vi "Z Stack Code.vi"() -> ()   [LabVIEW 2020]
uses:
  <vilib>/DAQmx/write.llb/DAQmx Write (Analog 1D Wfm NChan NSamp).vi
  <vilib>/DAQmx/create/channels.llb/DAQmx Create Channel (AO-Voltage-Basic).vi
  <vilib>/DAQmx/configure/timing.llb/DAQmx Timing (Use Waveform).vi
  <vilib>/DAQmx/miscellaneous.llb/DAQmx Fill In Error Info.vi
  <vilib>/Utility/file.llb/Read Delimited Spreadsheet (DBL).vi
  <vilib>/Analysis/polynomials.llb/Subtract Polynomials (DBL).vi
  <vilib>/measure/NI_MABase.lvlib
  <vilib>/Analysis/NI_AALPro.lvlib
panel:
  out "Waveform Graph":waveform(dbl)[](graph)=[{"t0"=timestamp(0 s since 1904-01-01), "dt"=0.0001, "Y"=array[10000 elements]}, {"t0"=timestamp(0 s since 1904-01-01), "dt"=0.0001, "Y"=array[10000 elements]}]
  out "dt":dbl=0.0001
  in  "file path (dialog if empty) 2":path=path "C:/Users/htm22/Downloads/Subtractfitvaluefromoutput.txt"
  out "x-y":dbl[](array[numeric])=[0.0, 0.0, 0.0, 0.0, 0.0, 0.0, 0.0, 0.0, 0.0, 0.0, 0.0, 0.0, 0.0, 0.0, 0.0, 0.0, 0.0, 0.0, 0.0, 0.0, 0.0, 0.0, 0.0, 0.0, 0.0, 0.0, 0.0, 0.0, 0.0, 0.0, 0.0, 0.0, 0.0, 0.0, 0.0, 0.0, 0.0, 0.0, 0.0, 0.0, 0.0, 0.0, 0.0, 0.0, 0.0, 0.0, 0.0, 0.0, 0.0, 0.0, 0.0, 0.0, 0.0, 0.0, 0.0, 0.0, 0.00936, -0.01208, 0.00648, -0.01496, 0.0036, 0.00216, -0.01928, -0.00072, -0.00216, -0.0036, -0.02504, 0.01352, 0.01208, -0.00936, 0.0092, 0.00776, -0.01368, -0.03512, -0.01656, -0.018, 0.00056, -0.00088, -0.02232, -0.00376, -0.0052, -0.02664, -0.02808, -0.00952, -0.01096, 0.0076, -0.01384, 0.00472, 0.00328, -0.01816, -0.0196, -0.02104, -0.02248, -0.00392, -0.00536, -0.0268, -0.00824, -0.00968, -0.01112, -0.01256, -0.014, 0.00456, 0.00312, 0.00168, 0.00024, -0.0212, -0.00264, -0.02408, -0.00552, -0.02696, -0.0084, -0.02984, 0.00872, 0.00728, -0.01416, -0.0356, -0.01704, 0.00152, 8e-05, -0.00136, -0.0028, -0.00424, -0.02568, -0.00712, -0.00856, -0.01, -0.01144, -0.03288, -0.03432, -0.01576, 0.0028, -0.01864, 0.01992, -0.02152, -0.02296, -0.0244, 0.01416, -0.00728, -0.00872, -0.01016, -0.0116, -0.01304, -0.01448, -0.01592, 0.00264, -0.0188, -0.02024, -0.00168, -0.00312, -0.04456, 0.014, -0.00744, -0.00888, 0.00968, -0.01176, 0.0068, -0.01464, -0.01608, -0.01752, 0.00104, -0.0004, -0.00184, -0.00328, -0.02472, -0.00616, -0.0076, -0.00904, -0.01048, -0.01192, -0.01336, -0.0148, -0.01624, -0.01768, -0.01912, -0.02056, -0.002, -0.00344, -0.02488, -0.00632, -0.02776, -0.0292, -0.03064, -0.01208, 0.00648, -0.01496, 0.0036, 0.00216, 0.00072, -0.00072, -0.02216, -0.0236, -0.00504, -0.00648, -0.00792, -0.00936, -0.0108, -0.01224, -0.01368, -0.01512, 0.00344, -0.018, 0.00056, -0.00088, -0.00232, -0.00376, -0.0052, -0.00664, -0.02808, -0.00952, 0.00904, -0.0124, -0.01384, -0.01528, -0.01672, -0.01816, -0.0196, -0.00104, -0.02248, -0.00392, 0.01464, -0.0068, -0.02824, 0.01032, -0.01112, 0.00744, -0.014, 0.00456, 0.00312, -0.01832, 0.00024, -0.0212, -0.02264, -0.00408, -0.00552, -0.02696, -0.0284, -0.00984, 0.00872, 0.00728, 0.00584, 0.0044, 0.00296, 0.00152, 8e-05, -0.02136, -0.0028, -0.02424, -0.00568, -0.00712, 0.01144, -0.01, -0.01144, -0.01288, 0.00568, -0.01576, -0.0172, 0.00136, -8e-05, -0.00152, -0.00296, 0.0156, -0.02584, -0.00728, -0.02872, -0.01016, -0.0116, -0.01304, 0.00552, -0.03592, -0.01736, -0.0188, -0.02024, -0.02168, -0.02312, -0.00456, -0.006, -0.00744, -0.00888, 0.00968, -0.01176, 0.0068, -0.01464, -0.01608, -0.01752, -0.01896, -0.0004, -0.00184, 0.01672, 0.01528, -0.00616, -0.0276, 0.01096, -0.01048, -0.01192, -0.01336, -0.0148, -0.01624, -0.01768, 0.00088, -0.02056, -0.022, -0.02344, -0.02488, 0.01368, -0.00776, -0.0092, -0.01064, -0.01208, 0.00648, -0.01496, -0.0364, -0.01784, 0.00072, -0.00072, -0.02216, -0.0036, -0.00504, -0.00648, -0.02792, -0.02936, 0.0092, 0.00776, 0.00632, -0.03512, 0.00344, -0.018, -0.01944, -0.00088, -0.00232, -0.00376, -0.0052, -0.02664, -0.00808, -0.00952, -0.01096, -0.0124, -0.01384, 0.00472, 0.00328, -0.01816, 0.0204, -0.00104, -0.00248, -0.00392, -0.00536, -0.0068, -0.02824, -0.02968, -0.01112, -0.01256, -0.014, -0.03544, 0.00312, 0.00168, 0.00024, -0.0012, -0.00264, -0.00408, -0.00552, -0.00696, -0.0084, 0.01016, -0.01128, -0.01272, 0.00584, -0.0156, -0.01704, 0.02152, 8e-05, -0.02136, -0.0028, -0.00424, -0.02568, -0.02712, 0.01144, 0.01, -0.01144, -0.01288, -0.01432, -0.01576, -0.0172, 0.00136, -0.02008, -0.00152, -0.02296, -0.0044, -0.02584, -0.00728, -0.02872, -0.01016, -0.0116, -0.01304, -0.01448, 0.00408, 0.00264, -0.0188, -0.02024, -0.00168, -0.02312, -0.02456, -0.006, -0.00744, -0.00888, -0.01032, -0.01176, -0.0132, -0.01464, -0.03608, 0.00248, 0.00104, -0.0204, 0.01816, -0.00328, -0.00472, -0.00616, -0.0076, -0.02904, -0.03048, -0.01192, -0.01336, -0.0148, 0.00376, -0.03768, -0.03912, -0.00056, -0.022, 0.01656, -0.00488, -0.00632, -0.00776, -0.0292, -0.01064, -0.01208, -0.01352, -0.01496, -0.0364, -0.01784, -0.01928, -0.02072, 0.01784, -0.0036, -0.02504, -0.00648, -0.00792, -0.02936, -0.0108, -0.01224, 0.00632, 0.00488, -0.01656, -0.038, 0.00056, -0.00088, -0.00232, -0.02376, -0.0052, -0.00664, -0.00808, -0.00952, -0.01096, -0.0324, -0.03384, -0.01528, -0.01672, -0.01816, -0.0196, -0.00104, -0.02248, -0.00392, -0.00536, -0.0068, -0.00824, -0.00968, 0.00888, -0.01256, -0.014, -0.01544, -0.01688, 0.00168, -0.01976, -0.0012, -0.00264, -0.00408, -0.02552, -0.00696, -0.0084, -0.00984, -0.01128, -0.01272, -0.01416, 0.0044, 0.00296, -0.01848, 8e-05, -0.00136, -0.0028, -0.02424, -0.00568, -0.00712, -0.00856, -0.01, -0.01144, -0.01288, -0.01432, -0.01576, 0.0028, -0.01864, -8e-05, -0.02152, -0.02296, -0.0044, -0.00584, -0.02728, -0.00872, -0.01016, -0.0116, -0.03304, -0.03448, -0.01592, -0.01736, -0.0188, -0.02024, -0.02168, -0.02312, -0.02456, -0.006, -0.02744, -0.00888, -0.03032, -0.01176, -0.0132, -0.01464, -0.01608, 0.00248, -0.01896, -0.0204, -0.02184, -0.02328, -0.00472, -0.00616, -0.0076, -0.00904, -0.01048, -0.01192, -0.01336, 0.0052, -0.01624, -0.01768, -0.01912, -0.02056, -0.022, -0.02344, -0.00488, -0.00632, -0.02776, -0.0292, 0.00936, -0.01208, -0.03352, 0.00504, 0.0036, -0.01784, -0.01928, -0.00072, -0.02216, -0.0236, -0.02504, -0.00648, -0.00792, -0.00936, -0.0308, -0.01224, 0.00632, -0.01512, -0.01656, -0.018, -0.01944, -0.02088, -0.00232, -0.00376, -0.0252, -0.00664, -0.00808, -0.00952, -0.01096, 0.0076, -0.01384, -0.01528, -0.01672, 0.00184, 0.0004, -0.00104, -0.02248, -0.02392, -0.02536, -0.0068, 0.01176, -0.00968, -0.01112, -0.01256, -0.014, -0.01544, 0.00312, -0.01832, -0.01976, -0.0212, -0.00264, -0.00408, -0.00552, -0.02696, -0.0084, -0.00984, 0.00872, -0.03272, 0.00584, -0.0156, -0.01704, -0.01848, -0.01992, -0.00136, -0.0028, -0.00424, -0.02568, -0.00712, -0.00856, -0.01, -0.01144, -0.01288, -0.01432, -0.01576, -0.0372, 0.00136, -0.02008, -0.02152, -0.02296, -0.0044, -0.02584, -0.00728, -0.00872, -0.03016, -0.0116, -0.03304, 0.00552, -0.03592, -0.01736, 0.0012, -0.00024, -0.02168, -0.02312, -0.02456, -0.006, -0.02744, -0.00888, -0.03032, -0.03176, -0.0332, -0.01464, -0.01608, -0.01752, 0.00104, -0.0004, -0.02184, -0.00328, -0.00472, -0.00616, -0.0076, -0.00904, -0.03048, -0.01192, -0.01336, -0.0148, -0.01624, -0.01768, -0.01912, -0.02056, -0.002, -0.02344, -0.00488, -0.00632, -0.02776, 0.0108, -0.01064, -0.01208, -0.01352, 0.00504, 0.0036, 0.00216, 0.00072, -0.02072, -0.02216, -0.0236, -0.02504, -0.00648, -0.00792, 0.01064, 0.0092, -0.01224, -0.01368, 0.00488, -0.01656, 0.002, 0.00056, -0.00088, -0.00232, -0.00376, -0.0252, -0.02664, -0.00808, -0.00952, -0.01096, -0.0124, -0.03384, 0.00472, -0.01672, -0.01816, -0.0196, -0.00104, -0.00248, 0.01608, -0.00536, -0.0068, -0.00824, -0.02968, 0.00888, 0.00744, -0.014, 0.00456, -0.01688, 0.00168, -0.01976, -0.0012, -0.00264, -0.00408, -0.00552, -0.00696, -0.0284, -0.00984, 0.00872, -0.01272, -0.01416, -0.0156, -0.01704, -0.01848, -0.01992, -0.00136, -0.0228, -0.00424, -0.00568, -0.00712, -0.00856, -0.01, -0.01144, -0.01288, -0.01432, 0.00424, 0.0028, 0.00136, -0.02008, -0.00152, -0.02296, -0.0044, -0.00584, -0.02728, -0.00872, -0.03016, -0.0316, -0.01304, 0.00552, -0.03592, -0.01736, -0.0188, -0.00024, -0.02168, -0.02312, 0.01544, -0.006, -0.00744, -0.02888, -0.01032, -0.01176, 0.0068, -0.01464, -0.01608, -0.01752, 0.00104, -0.0204, -0.00184, -0.00328, -0.00472, -0.02616, -0.0076, -0.02904, -0.01048, -0.01192, -0.01336, 0.0052, -0.01624, -0.01768, 0.00088, -0.02056, -0.022, -0.00344, -0.02488, -0.00632, -0.00776, -0.0092, 0.00936, -0.03208, 0.02648, -0.01496, 0.0036, -0.01784, -0.01928, -0.00072, -0.00216, -0.0036, -0.00504, -0.00648, -0.00792, -0.00936, 0.0092, -0.03224, -0.01368, -0.01512, -0.01656, 0.002, -0.01944, -0.02088, -0.00232, -0.00376, -0.0052, -0.00664, -0.00808, -0.00952, -0.01096, -0.0124, -0.01384, -0.01528, -0.01672, 0.00184, -0.0196, -0.04104, -0.02248, -0.00392, -0.00536, -0.0268, -0.00824, -0.00968, -0.01112, -0.01256, -0.014, 0.00456, -0.01688, -0.01832, -0.01976, -0.0012, -0.02264, -0.00408, -0.00552, 0.01304, 0.0116, -0.00984, -0.01128, -0.03272, -0.01416, -0.0156, 0.00296, 0.00152, 8e-05, -0.00136, -0.0228, -0.02424, -0.00568, -0.00712, -0.00856, -0.01, -0.01144, 0.00712, 0.00568, 0.00424, -0.0172, 0.00136, -0.02008, -0.02152, -0.02296, -0.0044, 0.01416, -0.00728, -0.02872, -0.01016, -0.0316, -0.01304, -0.01448, -0.01592, -0.01736, 0.0012, -0.02024, -0.02168, -0.00312, -0.00456, -0.006, -0.00744, 0.01112, -0.03032, -0.03176, -0.0332, -0.01464, -0.01608, -0.01752, 0.00104, -0.0004, -0.02184, -0.00328, 0.01528, -0.02616, -0.0076, -0.00904, -0.01048, -0.01192, -0.03336, -0.0148, -0.01624, -0.01768, 0.00088, -0.02056, -0.002, -0.00344, -0.02488, -0.02632, -0.02776, -0.0092, -0.01064, -0.01208, -0.01352, -0.01496, -0.0164, -0.01784, 0.00072, -0.00072, -0.04216, -0.0236, -0.00504, -0.00648, 0.01208, -0.00936, -0.0308, -0.03224, 0.00632, 0.00488, -0.01656, 0.002, 0.00056, -0.00088, -0.02232, -0.00376, -0.0052, -0.00664, -0.02808, -0.00952, -0.01096, -0.0124, -0.01384, -0.01528, -0.01672, -0.01816, 0.0004, -0.02104, -0.02248, -0.02392, -0.02536, -0.0068, -0.00824, -0.00968, 0.00888, -0.01256, -0.014, -0.01544, 0.00312, -0.03832, 0.00024, -0.0012, -0.00264, -0.02408, -0.00552, -0.02696, -0.0284, -0.00984, 0.00872, -0.01272, -0.01416, -0.0356, 0.00296, -0.01848, 8e-05, -0.00136, -0.0028, -0.02424, -0.02568, -0.00712, -0.00856]
  out "Signal - Fit":dbl[](graph)=[0.0, 0.0, 0.0, 0.0, 0.0, 0.0, 0.0, 0.0, 0.0, 0.0, 0.0, 0.0, 0.0, 0.0, 0.0, 0.0, 0.0, 0.0, 0.0, 0.0, 0.0, 0.0, 0.0, 0.0, 0.0, 0.0, 0.0, 0.0, 0.0, 0.0, 0.0, 0.0, 0.0, 0.0, 0.0, 0.0, 0.0, 0.0, 0.0, 0.0, 0.0, 0.0, 0.0, 0.0, 0.0, 0.0, 0.0, 0.0, 0.0, 0.0, 0.0, 0.0, 0.0, 0.0, 0.0, 0.0, 0.00936, -0.01208, 0.00648, -0.01496, 0.0036, 0.00216, -0.01928, -0.00072, -0.00216, -0.0036, -0.02504, 0.01352, 0.01208, -0.00936, 0.0092, 0.00776, -0.01368, -0.03512, -0.01656, -0.018, 0.00056, -0.00088, -0.02232, -0.00376, -0.0052, -0.02664, -0.02808, -0.00952, -0.01096, 0.0076, -0.01384, 0.00472, 0.00328, -0.01816, -0.0196, -0.02104, -0.02248, -0.00392, -0.00536, -0.0268, -0.00824, -0.00968, -0.01112, -0.01256, -0.014, 0.00456, 0.00312, 0.00168, 0.00024, -0.0212, -0.00264, -0.02408, -0.00552, -0.02696, -0.0084, -0.02984, 0.00872, 0.00728, -0.01416, -0.0356, -0.01704, 0.00152, 8e-05, -0.00136, -0.0028, -0.00424, -0.02568, -0.00712, -0.00856, -0.01, -0.01144, -0.03288, -0.03432, -0.01576, 0.0028, -0.01864, 0.01992, -0.02152, -0.02296, -0.0244, 0.01416, -0.00728, -0.00872, -0.01016, -0.0116, -0.01304, -0.01448, -0.01592, 0.00264, -0.0188, -0.02024, -0.00168, -0.00312, -0.04456, 0.014, -0.00744, -0.00888, 0.00968, -0.01176, 0.0068, -0.01464, -0.01608, -0.01752, 0.00104, -0.0004, -0.00184, -0.00328, -0.02472, -0.00616, -0.0076, -0.00904, -0.01048, -0.01192, -0.01336, -0.0148, -0.01624, -0.01768, -0.01912, -0.02056, -0.002, -0.00344, -0.02488, -0.00632, -0.02776, -0.0292, -0.03064, -0.01208, 0.00648, -0.01496, 0.0036, 0.00216, 0.00072, -0.00072, -0.02216, -0.0236, -0.00504, -0.00648, -0.00792, -0.00936, -0.0108, -0.01224, -0.01368, -0.01512, 0.00344, -0.018, 0.00056, -0.00088, -0.00232, -0.00376, -0.0052, -0.00664, -0.02808, -0.00952, 0.00904, -0.0124, -0.01384, -0.01528, -0.01672, -0.01816, -0.0196, -0.00104, -0.02248, -0.00392, 0.01464, -0.0068, -0.02824, 0.01032, -0.01112, 0.00744, -0.014, 0.00456, 0.00312, -0.01832, 0.00024, -0.0212, -0.02264, -0.00408, -0.00552, -0.02696, -0.0284, -0.00984, 0.00872, 0.00728, 0.00584, 0.0044, 0.00296, 0.00152, 8e-05, -0.02136, -0.0028, -0.02424, -0.00568, -0.00712, 0.01144, -0.01, -0.01144, -0.01288, 0.00568, -0.01576, -0.0172, 0.00136, -8e-05, -0.00152, -0.00296, 0.0156, -0.02584, -0.00728, -0.02872, -0.01016, -0.0116, -0.01304, 0.00552, -0.03592, -0.01736, -0.0188, -0.02024, -0.02168, -0.02312, -0.00456, -0.006, -0.00744, -0.00888, 0.00968, -0.01176, 0.0068, -0.01464, -0.01608, -0.01752, -0.01896, -0.0004, -0.00184, 0.01672, 0.01528, -0.00616, -0.0276, 0.01096, -0.01048, -0.01192, -0.01336, -0.0148, -0.01624, -0.01768, 0.00088, -0.02056, -0.022, -0.02344, -0.02488, 0.01368, -0.00776, -0.0092, -0.01064, -0.01208, 0.00648, -0.01496, -0.0364, -0.01784, 0.00072, -0.00072, -0.02216, -0.0036, -0.00504, -0.00648, -0.02792, -0.02936, 0.0092, 0.00776, 0.00632, -0.03512, 0.00344, -0.018, -0.01944, -0.00088, -0.00232, -0.00376, -0.0052, -0.02664, -0.00808, -0.00952, -0.01096, -0.0124, -0.01384, 0.00472, 0.00328, -0.01816, 0.0204, -0.00104, -0.00248, -0.00392, -0.00536, -0.0068, -0.02824, -0.02968, -0.01112, -0.01256, -0.014, -0.03544, 0.00312, 0.00168, 0.00024, -0.0012, -0.00264, -0.00408, -0.00552, -0.00696, -0.0084, 0.01016, -0.01128, -0.01272, 0.00584, -0.0156, -0.01704, 0.02152, 8e-05, -0.02136, -0.0028, -0.00424, -0.02568, -0.02712, 0.01144, 0.01, -0.01144, -0.01288, -0.01432, -0.01576, -0.0172, 0.00136, -0.02008, -0.00152, -0.02296, -0.0044, -0.02584, -0.00728, -0.02872, -0.01016, -0.0116, -0.01304, -0.01448, 0.00408, 0.00264, -0.0188, -0.02024, -0.00168, -0.02312, -0.02456, -0.006, -0.00744, -0.00888, -0.01032, -0.01176, -0.0132, -0.01464, -0.03608, 0.00248, 0.00104, -0.0204, 0.01816, -0.00328, -0.00472, -0.00616, -0.0076, -0.02904, -0.03048, -0.01192, -0.01336, -0.0148, 0.00376, -0.03768, -0.03912, -0.00056, -0.022, 0.01656, -0.00488, -0.00632, -0.00776, -0.0292, -0.01064, -0.01208, -0.01352, -0.01496, -0.0364, -0.01784, -0.01928, -0.02072, 0.01784, -0.0036, -0.02504, -0.00648, -0.00792, -0.02936, -0.0108, -0.01224, 0.00632, 0.00488, -0.01656, -0.038, 0.00056, -0.00088, -0.00232, -0.02376, -0.0052, -0.00664, -0.00808, -0.00952, -0.01096, -0.0324, -0.03384, -0.01528, -0.01672, -0.01816, -0.0196, -0.00104, -0.02248, -0.00392, -0.00536, -0.0068, -0.00824, -0.00968, 0.00888, -0.01256, -0.014, -0.01544, -0.01688, 0.00168, -0.01976, -0.0012, -0.00264, -0.00408, -0.02552, -0.00696, -0.0084, -0.00984, -0.01128, -0.01272, -0.01416, 0.0044, 0.00296, -0.01848, 8e-05, -0.00136, -0.0028, -0.02424, -0.00568, -0.00712, -0.00856, -0.01, -0.01144, -0.01288, -0.01432, -0.01576, 0.0028, -0.01864, -8e-05, -0.02152, -0.02296, -0.0044, -0.00584, -0.02728, -0.00872, -0.01016, -0.0116, -0.03304, -0.03448, -0.01592, -0.01736, -0.0188, -0.02024, -0.02168, -0.02312, -0.02456, -0.006, -0.02744, -0.00888, -0.03032, -0.01176, -0.0132, -0.01464, -0.01608, 0.00248, -0.01896, -0.0204, -0.02184, -0.02328, -0.00472, -0.00616, -0.0076, -0.00904, -0.01048, -0.01192, -0.01336, 0.0052, -0.01624, -0.01768, -0.01912, -0.02056, -0.022, -0.02344, -0.00488, -0.00632, -0.02776, -0.0292, 0.00936, -0.01208, -0.03352, 0.00504, 0.0036, -0.01784, -0.01928, -0.00072, -0.02216, -0.0236, -0.02504, -0.00648, -0.00792, -0.00936, -0.0308, -0.01224, 0.00632, -0.01512, -0.01656, -0.018, -0.01944, -0.02088, -0.00232, -0.00376, -0.0252, -0.00664, -0.00808, -0.00952, -0.01096, 0.0076, -0.01384, -0.01528, -0.01672, 0.00184, 0.0004, -0.00104, -0.02248, -0.02392, -0.02536, -0.0068, 0.01176, -0.00968, -0.01112, -0.01256, -0.014, -0.01544, 0.00312, -0.01832, -0.01976, -0.0212, -0.00264, -0.00408, -0.00552, -0.02696, -0.0084, -0.00984, 0.00872, -0.03272, 0.00584, -0.0156, -0.01704, -0.01848, -0.01992, -0.00136, -0.0028, -0.00424, -0.02568, -0.00712, -0.00856, -0.01, -0.01144, -0.01288, -0.01432, -0.01576, -0.0372, 0.00136, -0.02008, -0.02152, -0.02296, -0.0044, -0.02584, -0.00728, -0.00872, -0.03016, -0.0116, -0.03304, 0.00552, -0.03592, -0.01736, 0.0012, -0.00024, -0.02168, -0.02312, -0.02456, -0.006, -0.02744, -0.00888, -0.03032, -0.03176, -0.0332, -0.01464, -0.01608, -0.01752, 0.00104, -0.0004, -0.02184, -0.00328, -0.00472, -0.00616, -0.0076, -0.00904, -0.03048, -0.01192, -0.01336, -0.0148, -0.01624, -0.01768, -0.01912, -0.02056, -0.002, -0.02344, -0.00488, -0.00632, -0.02776, 0.0108, -0.01064, -0.01208, -0.01352, 0.00504, 0.0036, 0.00216, 0.00072, -0.02072, -0.02216, -0.0236, -0.02504, -0.00648, -0.00792, 0.01064, 0.0092, -0.01224, -0.01368, 0.00488, -0.01656, 0.002, 0.00056, -0.00088, -0.00232, -0.00376, -0.0252, -0.02664, -0.00808, -0.00952, -0.01096, -0.0124, -0.03384, 0.00472, -0.01672, -0.01816, -0.0196, -0.00104, -0.00248, 0.01608, -0.00536, -0.0068, -0.00824, -0.02968, 0.00888, 0.00744, -0.014, 0.00456, -0.01688, 0.00168, -0.01976, -0.0012, -0.00264, -0.00408, -0.00552, -0.00696, -0.0284, -0.00984, 0.00872, -0.01272, -0.01416, -0.0156, -0.01704, -0.01848, -0.01992, -0.00136, -0.0228, -0.00424, -0.00568, -0.00712, -0.00856, -0.01, -0.01144, -0.01288, -0.01432, 0.00424, 0.0028, 0.00136, -0.02008, -0.00152, -0.02296, -0.0044, -0.00584, -0.02728, -0.00872, -0.03016, -0.0316, -0.01304, 0.00552, -0.03592, -0.01736, -0.0188, -0.00024, -0.02168, -0.02312, 0.01544, -0.006, -0.00744, -0.02888, -0.01032, -0.01176, 0.0068, -0.01464, -0.01608, -0.01752, 0.00104, -0.0204, -0.00184, -0.00328, -0.00472, -0.02616, -0.0076, -0.02904, -0.01048, -0.01192, -0.01336, 0.0052, -0.01624, -0.01768, 0.00088, -0.02056, -0.022, -0.00344, -0.02488, -0.00632, -0.00776, -0.0092, 0.00936, -0.03208, 0.02648, -0.01496, 0.0036, -0.01784, -0.01928, -0.00072, -0.00216, -0.0036, -0.00504, -0.00648, -0.00792, -0.00936, 0.0092, -0.03224, -0.01368, -0.01512, -0.01656, 0.002, -0.01944, -0.02088, -0.00232, -0.00376, -0.0052, -0.00664, -0.00808, -0.00952, -0.01096, -0.0124, -0.01384, -0.01528, -0.01672, 0.00184, -0.0196, -0.04104, -0.02248, -0.00392, -0.00536, -0.0268, -0.00824, -0.00968, -0.01112, -0.01256, -0.014, 0.00456, -0.01688, -0.01832, -0.01976, -0.0012, -0.02264, -0.00408, -0.00552, 0.01304, 0.0116, -0.00984, -0.01128, -0.03272, -0.01416, -0.0156, 0.00296, 0.00152, 8e-05, -0.00136, -0.0228, -0.02424, -0.00568, -0.00712, -0.00856, -0.01, -0.01144, 0.00712, 0.00568, 0.00424, -0.0172, 0.00136, -0.02008, -0.02152, -0.02296, -0.0044, 0.01416, -0.00728, -0.02872, -0.01016, -0.0316, -0.01304, -0.01448, -0.01592, -0.01736, 0.0012, -0.02024, -0.02168, -0.00312, -0.00456, -0.006, -0.00744, 0.01112, -0.03032, -0.03176, -0.0332, -0.01464, -0.01608, -0.01752, 0.00104, -0.0004, -0.02184, -0.00328, 0.01528, -0.02616, -0.0076, -0.00904, -0.01048, -0.01192, -0.03336, -0.0148, -0.01624, -0.01768, 0.00088, -0.02056, -0.002, -0.00344, -0.02488, -0.02632, -0.02776, -0.0092, -0.01064, -0.01208, -0.01352, -0.01496, -0.0164, -0.01784, 0.00072, -0.00072, -0.04216, -0.0236, -0.00504, -0.00648, 0.01208, -0.00936, -0.0308, -0.03224, 0.00632, 0.00488, -0.01656, 0.002, 0.00056, -0.00088, -0.02232, -0.00376, -0.0052, -0.00664, -0.02808, -0.00952, -0.01096, -0.0124, -0.01384, -0.01528, -0.01672, -0.01816, 0.0004, -0.02104, -0.02248, -0.02392, -0.02536, -0.0068, -0.00824, -0.00968, 0.00888, -0.01256, -0.014, -0.01544, 0.00312, -0.03832, 0.00024, -0.0012, -0.00264, -0.02408, -0.00552, -0.02696, -0.0284, -0.00984, 0.00872, -0.01272, -0.01416, -0.0356, 0.00296, -0.01848, 8e-05, -0.00136, -0.0028, -0.02424, -0.02568, -0.00712, -0.00856]
  out "Array":dbl[](array[numeric])=[0.0, 0.001, 0.002, 0.003, 0.004, 0.005, 0.006, 0.007, 0.008, 0.009, 0.01, 0.011, 0.012, 0.013, 0.014, 0.015, 0.016, 0.017, 0.018, 0.019, 0.02, 0.021, 0.022, 0.023, 0.024, 0.025, 0.026, 0.027, 0.028, 0.029, 0.03, 0.031, 0.032, 0.033, 0.034, 0.035, 0.036, 0.037, 0.038, 0.039, 0.04, 0.041, 0.042, 0.043, 0.044, 0.045, 0.046, 0.047, 0.048, 0.049, 0.05, 0.051, 0.052, 0.053, 0.054, 0.055, 0.056, 0.057, 0.058, 0.059, 0.06, 0.061, 0.062, 0.063, 0.064, 0.065, 0.066, 0.067, 0.068, 0.069, 0.07, 0.071, 0.072, 0.073, 0.074, 0.075, 0.076, 0.077, 0.078, 0.079, 0.08, 0.081, 0.082, 0.083, 0.084, 0.085, 0.086, 0.087, 0.088, 0.089, 0.09, 0.091, 0.092, 0.093, 0.094, 0.095, 0.096, 0.097, 0.098, 0.099, 0.1, 0.101, 0.102, 0.103, 0.104, 0.105, 0.106, 0.107, 0.108, 0.109, 0.11, 0.111, 0.112, 0.113, 0.114, 0.115, 0.116, 0.117, 0.118, 0.119, 0.12, 0.121, 0.122, 0.123, 0.124, 0.125, 0.126, 0.127, 0.128, 0.129, 0.13, 0.131, 0.132, 0.133, 0.134, 0.135, 0.136, 0.137, 0.138, 0.139, 0.14, 0.141, 0.142, 0.143, 0.144, 0.145, 0.146, 0.147, 0.148, 0.149, 0.15, 0.151, 0.152, 0.153, 0.154, 0.155, 0.156, 0.157, 0.158, 0.159, 0.16, 0.161, 0.162, 0.163, 0.164, 0.165, 0.166, 0.167, 0.168, 0.169, 0.17, 0.171, 0.172, 0.173, 0.174, 0.175, 0.176, 0.177, 0.178, 0.179, 0.18, 0.181, 0.182, 0.183, 0.184, 0.185, 0.186, 0.187, 0.188, 0.189, 0.19, 0.191, 0.192, 0.193, 0.194, 0.195, 0.196, 0.197, 0.198, 0.199, 0.2, 0.201, 0.202, 0.203, 0.204, 0.205, 0.206, 0.207, 0.208, 0.209, 0.21, 0.211, 0.212, 0.213, 0.214, 0.215, 0.216, 0.217, 0.218, 0.219, 0.22, 0.221, 0.222, 0.223, 0.224, 0.225, 0.226, 0.227, 0.228, 0.229, 0.23, 0.231, 0.232, 0.233, 0.234, 0.235, 0.236, 0.237, 0.238, 0.239, 0.24, 0.241, 0.242, 0.243, 0.244, 0.245, 0.246, 0.247, 0.248, 0.249, 0.25, 0.251, 0.252, 0.253, 0.254, 0.255, 0.256, 0.257, 0.258, 0.259, 0.26, 0.261, 0.262, 0.263, 0.264, 0.265, 0.266, 0.267, 0.268, 0.269, 0.27, 0.271, 0.272, 0.273, 0.274, 0.275, 0.276, 0.277, 0.278, 0.279, 0.28, 0.281, 0.282, 0.283, 0.284, 0.285, 0.286, 0.287, 0.288, 0.289, 0.29, 0.291, 0.292, 0.293, 0.294, 0.295, 0.296, 0.297, 0.298, 0.299, 0.3, 0.301, 0.302, 0.303, 0.304, 0.305, 0.306, 0.307, 0.308, 0.309, 0.31, 0.311, 0.312, 0.313, 0.314, 0.315, 0.316, 0.317, 0.318, 0.319, 0.32, 0.321, 0.322, 0.323, 0.324, 0.325, 0.326, 0.327, 0.328, 0.329, 0.33, 0.331, 0.332, 0.333, 0.334, 0.335, 0.336, 0.337, 0.338, 0.339, 0.34, 0.341, 0.342, 0.343, 0.344, 0.345, 0.346, 0.347, 0.348, 0.349, 0.35, 0.351, 0.352, 0.353, 0.354, 0.355, 0.356, 0.357, 0.358, 0.359, 0.36, 0.361, 0.362, 0.363, 0.364, 0.365, 0.366, 0.367, 0.368, 0.369, 0.37, 0.371, 0.372, 0.373, 0.374, 0.375, 0.376, 0.377, 0.378, 0.379, 0.38, 0.381, 0.382, 0.383, 0.384, 0.385, 0.386, 0.387, 0.388, 0.389, 0.39, 0.391, 0.392, 0.393, 0.394, 0.395, 0.396, 0.397, 0.398, 0.399, 0.4, 0.401, 0.402, 0.403, 0.404, 0.405, 0.406, 0.407, 0.408, 0.409, 0.41, 0.411, 0.412, 0.413, 0.414, 0.415, 0.416, 0.417, 0.418, 0.419, 0.42, 0.421, 0.422, 0.423, 0.424, 0.425, 0.426, 0.427, 0.428, 0.429, 0.43, 0.431, 0.432, 0.433, 0.434, 0.435, 0.436, 0.437, 0.438, 0.439, 0.44, 0.441, 0.442, 0.443, 0.444, 0.445, 0.446, 0.447, 0.448, 0.449, 0.45, 0.451, 0.452, 0.453, 0.454, 0.455, 0.456, 0.457, 0.458, 0.459, 0.46, 0.461, 0.462, 0.463, 0.464, 0.465, 0.466, 0.467, 0.468, 0.469, 0.47, 0.471, 0.472, 0.473, 0.474, 0.475, 0.476, 0.477, 0.478, 0.479, 0.48, 0.481, 0.482, 0.483, 0.484, 0.485, 0.486, 0.487, 0.488, 0.489, 0.49, 0.491, 0.492, 0.493, 0.494, 0.495, 0.496, 0.497, 0.498, 0.499, 0.5, 0.501, 0.502, 0.503, 0.504, 0.505, 0.506, 0.507, 0.508, 0.509, 0.51, 0.511, 0.512, 0.513, 0.514, 0.515, 0.516, 0.517, 0.518, 0.519, 0.52, 0.521, 0.522, 0.523, 0.524, 0.525, 0.526, 0.527, 0.528, 0.529, 0.53, 0.531, 0.532, 0.533, 0.534, 0.535, 0.536, 0.537, 0.538, 0.539, 0.54, 0.541, 0.542, 0.543, 0.544, 0.545, 0.546, 0.547, 0.548, 0.549, 0.55, 0.551, 0.552, 0.553, 0.554, 0.555, 0.556, 0.557, 0.558, 0.559, 0.56, 0.561, 0.562, 0.563, 0.564, 0.565, 0.566, 0.567, 0.568, 0.569, 0.57, 0.571, 0.572, 0.573, 0.574, 0.575, 0.576, 0.577, 0.578, 0.579, 0.58, 0.581, 0.582, 0.583, 0.584, 0.585, 0.586, 0.587, 0.588, 0.589, 0.59, 0.591, 0.592, 0.593, 0.594, 0.595, 0.596, 0.597, 0.598, 0.599, 0.6, 0.601, 0.602, 0.603, 0.604, 0.605, 0.606, 0.607, 0.608, 0.609, 0.61, 0.611, 0.612, 0.613, 0.614, 0.615, 0.616, 0.617, 0.618, 0.619, 0.62, 0.621, 0.622, 0.623, 0.624, 0.625, 0.626, 0.627, 0.628, 0.629, 0.63, 0.631, 0.632, 0.633, 0.634, 0.635, 0.636, 0.637, 0.638, 0.639, 0.64, 0.641, 0.642, 0.643, 0.644, 0.645, 0.646, 0.647, 0.648, 0.649, 0.65, 0.651, 0.652, 0.653, 0.654, 0.655, 0.656, 0.657, 0.658, 0.659, 0.66, 0.661, 0.662, 0.663, 0.664, 0.665, 0.666, 0.667, 0.668, 0.669, 0.67, 0.671, 0.672, 0.673, 0.674, 0.675, 0.676, 0.677, 0.678, 0.679, 0.68, 0.681, 0.682, 0.683, 0.684, 0.685, 0.686, 0.687, 0.688, 0.689, 0.69, 0.691, 0.692, 0.693, 0.694, 0.695, 0.696, 0.697, 0.698, 0.699, 0.7, 0.701, 0.702, 0.703, 0.704, 0.705, 0.706, 0.707, 0.708, 0.709, 0.71, 0.711, 0.712, 0.713, 0.714, 0.715, 0.716, 0.717, 0.718, 0.719, 0.72, 0.721, 0.722, 0.723, 0.724, 0.725, 0.726, 0.727, 0.728, 0.729, 0.73, 0.731, 0.732, 0.733, 0.734, 0.735, 0.736, 0.737, 0.738, 0.739, 0.74, 0.741, 0.742, 0.743, 0.744, 0.745, 0.746, 0.747, 0.748, 0.749, 0.75, 0.751, 0.752, 0.753, 0.754, 0.755, 0.756, 0.757, 0.758, 0.759, 0.76, 0.761, 0.762, 0.763, 0.764, 0.765, 0.766, 0.767, 0.768, 0.769, 0.77, 0.771, 0.772, 0.773, 0.774, 0.775, 0.776, 0.777, 0.778, 0.779, 0.78, 0.781, 0.782, 0.783, 0.784, 0.785, 0.786, 0.787, 0.788, 0.789, 0.79, 0.791, 0.792, 0.793, 0.794, 0.795, 0.796, 0.797, 0.798, 0.799, 0.8, 0.801, 0.802, 0.803, 0.804, 0.805, 0.806, 0.807, 0.808, 0.809, 0.81, 0.811, 0.812, 0.813, 0.814, 0.815, 0.816, 0.817, 0.818, 0.819, 0.82, 0.821, 0.822, 0.823, 0.824, 0.825, 0.826, 0.827, 0.828, 0.829, 0.83, 0.831, 0.832, 0.833, 0.834, 0.835, 0.836, 0.837, 0.838, 0.839, 0.84, 0.841, 0.842, 0.843, 0.844, 0.845, 0.846, 0.847, 0.848, 0.849, 0.85, 0.851, 0.852, 0.853, 0.854, 0.855, 0.856, 0.857, 0.858, 0.859, 0.86, 0.861, 0.862, 0.863, 0.864, 0.865, 0.866, 0.867, 0.868, 0.869, 0.87, 0.871, 0.872, 0.873, 0.874, 0.875, 0.876, 0.877, 0.878, 0.879, 0.88, 0.881, 0.882, 0.883, 0.884, 0.885, 0.886, 0.887, 0.888, 0.889, 0.89, 0.891, 0.892, 0.893, 0.894, 0.895, 0.896, 0.897, 0.898, 0.899, 0.9, 0.901, 0.902, 0.903, 0.904, 0.905, 0.906, 0.907, 0.908, 0.909, 0.91, 0.911, 0.912, 0.913, 0.914, 0.915, 0.916, 0.917, 0.918, 0.919, 0.92, 0.921, 0.922, 0.923, 0.924, 0.925, 0.926, 0.927, 0.928, 0.929, 0.93, 0.931, 0.932, 0.933, 0.934, 0.935, 0.936, 0.937, 0.938, 0.939, 0.94, 0.941, 0.942, 0.943, 0.944, 0.945, 0.946, 0.947, 0.948, 0.949, 0.95, 0.951, 0.952, 0.953, 0.954, 0.955, 0.956, 0.957, 0.958, 0.959, 0.96, 0.961, 0.962, 0.963, 0.964, 0.965, 0.966, 0.967, 0.968, 0.969, 0.97, 0.971, 0.972, 0.973, 0.974, 0.975, 0.976, 0.977, 0.978, 0.979, 0.98, 0.981, 0.982, 0.983, 0.984, 0.985, 0.986, 0.987, 0.988, 0.989, 0.99, 0.991, 0.992, 0.993, 0.994, 0.995, 0.996, 0.997, 0.998, 0.999]
  out "all rows 2":dbl[][](array[numeric])=[[0.0], [0.0], [0.0], [0.0], [0.0], [0.0], [0.0], [0.0], [0.0], [0.0], [0.0], [0.0], [0.0], [0.0], [0.0], [0.0], [0.0], [0.0], [0.0], [0.0], [0.0], [0.0], [0.0], [0.0], [0.0], [0.0], [0.0], [0.0], [0.0], [0.0], [0.0], [0.0], [0.0], [0.0], [0.0], [0.0], [0.0], [0.0], [0.0], [0.0], [0.0], [0.0], [0.0], [0.0], [0.0], [0.0], [0.0], [0.0], [0.0], [0.0], [0.0], [0.0], [0.0], [0.0], [0.0], [0.0], [0.00936], [-0.01208], [0.00648], [-0.01496], [0.0036], [0.00216], [-0.01928], [-0.00072], [-0.00216], [-0.0036], [-0.02504], [0.01352], [0.01208], [-0.00936], [0.0092], [0.00776], [-0.01368], [-0.03512], [-0.01656], [-0.018], [0.00056], [-0.00088], [-0.02232], [-0.00376], [-0.0052], [-0.02664], [-0.02808], [-0.00952], [-0.01096], [0.0076], [-0.01384], [0.00472], [0.00328], [-0.01816], [-0.0196], [-0.02104], [-0.02248], [-0.00392], [-0.00536], [-0.0268], [-0.00824], [-0.00968], [-0.01112], [-0.01256], [-0.014], [0.00456], [0.00312], [0.00168], [0.00024], [-0.0212], [-0.00264], [-0.02408], [-0.00552], [-0.02696], [-0.0084], [-0.02984], [0.00872], [0.00728], [-0.01416], [-0.0356], [-0.01704], [0.00152], [8e-05], [-0.00136], [-0.0028], [-0.00424], [-0.02568], [-0.00712], [-0.00856], [-0.01], [-0.01144], [-0.03288], [-0.03432], [-0.01576], [0.0028], [-0.01864], [0.01992], [-0.02152], [-0.02296], [-0.0244], [0.01416], [-0.00728], [-0.00872], [-0.01016], [-0.0116], [-0.01304], [-0.01448], [-0.01592], [0.00264], [-0.0188], [-0.02024], [-0.00168], [-0.00312], [-0.04456], [0.014], [-0.00744], [-0.00888], [0.00968], [-0.01176], [0.0068], [-0.01464], [-0.01608], [-0.01752], [0.00104], [-0.0004], [-0.00184], [-0.00328], [-0.02472], [-0.00616], [-0.0076], [-0.00904], [-0.01048], [-0.01192], [-0.01336], [-0.0148], [-0.01624], [-0.01768], [-0.01912], [-0.02056], [-0.002], [-0.00344], [-0.02488], [-0.00632], [-0.02776], [-0.0292], [-0.03064], [-0.01208], [0.00648], [-0.01496], [0.0036], [0.00216], [0.00072], [-0.00072], [-0.02216], [-0.0236], [-0.00504], [-0.00648], [-0.00792], [-0.00936], [-0.0108], [-0.01224], [-0.01368], [-0.01512], [0.00344], [-0.018], [0.00056], [-0.00088], [-0.00232], [-0.00376], [-0.0052], [-0.00664], [-0.02808], [-0.00952], [0.00904], [-0.0124], [-0.01384], [-0.01528], [-0.01672], [-0.01816], [-0.0196], [-0.00104], [-0.02248], [-0.00392], [0.01464], [-0.0068], [-0.02824], [0.01032], [-0.01112], [0.00744], [-0.014], [0.00456], [0.00312], [-0.01832], [0.00024], [-0.0212], [-0.02264], [-0.00408], [-0.00552], [-0.02696], [-0.0284], [-0.00984], [0.00872], [0.00728], [0.00584], [0.0044], [0.00296], [0.00152], [8e-05], [-0.02136], [-0.0028], [-0.02424], [-0.00568], [-0.00712], [0.01144], [-0.01], [-0.01144], [-0.01288], [0.00568], [-0.01576], [-0.0172], [0.00136], [-8e-05], [-0.00152], [-0.00296], [0.0156], [-0.02584], [-0.00728], [-0.02872], [-0.01016], [-0.0116], [-0.01304], [0.00552], [-0.03592], [-0.01736], [-0.0188], [-0.02024], [-0.02168], [-0.02312], [-0.00456], [-0.006], [-0.00744], [-0.00888], [0.00968], [-0.01176], [0.0068], [-0.01464], [-0.01608], [-0.01752], [-0.01896], [-0.0004], [-0.00184], [0.01672], [0.01528], [-0.00616], [-0.0276], [0.01096], [-0.01048], [-0.01192], [-0.01336], [-0.0148], [-0.01624], [-0.01768], [0.00088], [-0.02056], [-0.022], [-0.02344], [-0.02488], [0.01368], [-0.00776], [-0.0092], [-0.01064], [-0.01208], [0.00648], [-0.01496], [-0.0364], [-0.01784], [0.00072], [-0.00072], [-0.02216], [-0.0036], [-0.00504], [-0.00648], [-0.02792], [-0.02936], [0.0092], [0.00776], [0.00632], [-0.03512], [0.00344], [-0.018], [-0.01944], [-0.00088], [-0.00232], [-0.00376], [-0.0052], [-0.02664], [-0.00808], [-0.00952], [-0.01096], [-0.0124], [-0.01384], [0.00472], [0.00328], [-0.01816], [0.0204], [-0.00104], [-0.00248], [-0.00392], [-0.00536], [-0.0068], [-0.02824], [-0.02968], [-0.01112], [-0.01256], [-0.014], [-0.03544], [0.00312], [0.00168], [0.00024], [-0.0012], [-0.00264], [-0.00408], [-0.00552], [-0.00696], [-0.0084], [0.01016], [-0.01128], [-0.01272], [0.00584], [-0.0156], [-0.01704], [0.02152], [8e-05], [-0.02136], [-0.0028], [-0.00424], [-0.02568], [-0.02712], [0.01144], [0.01], [-0.01144], [-0.01288], [-0.01432], [-0.01576], [-0.0172], [0.00136], [-0.02008], [-0.00152], [-0.02296], [-0.0044], [-0.02584], [-0.00728], [-0.02872], [-0.01016], [-0.0116], [-0.01304], [-0.01448], [0.00408], [0.00264], [-0.0188], [-0.02024], [-0.00168], [-0.02312], [-0.02456], [-0.006], [-0.00744], [-0.00888], [-0.01032], [-0.01176], [-0.0132], [-0.01464], [-0.03608], [0.00248], [0.00104], [-0.0204], [0.01816], [-0.00328], [-0.00472], [-0.00616], [-0.0076], [-0.02904], [-0.03048], [-0.01192], [-0.01336], [-0.0148], [0.00376], [-0.03768], [-0.03912], [-0.00056], [-0.022], [0.01656], [-0.00488], [-0.00632], [-0.00776], [-0.0292], [-0.01064], [-0.01208], [-0.01352], [-0.01496], [-0.0364], [-0.01784], [-0.01928], [-0.02072], [0.01784], [-0.0036], [-0.02504], [-0.00648], [-0.00792], [-0.02936], [-0.0108], [-0.01224], [0.00632], [0.00488], [-0.01656], [-0.038], [0.00056], [-0.00088], [-0.00232], [-0.02376], [-0.0052], [-0.00664], [-0.00808], [-0.00952], [-0.01096], [-0.0324], [-0.03384], [-0.01528], [-0.01672], [-0.01816], [-0.0196], [-0.00104], [-0.02248], [-0.00392], [-0.00536], [-0.0068], [-0.00824], [-0.00968], [0.00888], [-0.01256], [-0.014], [-0.01544], [-0.01688], [0.00168], [-0.01976], [-0.0012], [-0.00264], [-0.00408], [-0.02552], [-0.00696], [-0.0084], [-0.00984], [-0.01128], [-0.01272], [-0.01416], [0.0044], [0.00296], [-0.01848], [8e-05], [-0.00136], [-0.0028], [-0.02424], [-0.00568], [-0.00712], [-0.00856], [-0.01], [-0.01144], [-0.01288], [-0.01432], [-0.01576], [0.0028], [-0.01864], [-8e-05], [-0.02152], [-0.02296], [-0.0044], [-0.00584], [-0.02728], [-0.00872], [-0.01016], [-0.0116], [-0.03304], [-0.03448], [-0.01592], [-0.01736], [-0.0188], [-0.02024], [-0.02168], [-0.02312], [-0.02456], [-0.006], [-0.02744], [-0.00888], [-0.03032], [-0.01176], [-0.0132], [-0.01464], [-0.01608], [0.00248], [-0.01896], [-0.0204], [-0.02184], [-0.02328], [-0.00472], [-0.00616], [-0.0076], [-0.00904], [-0.01048], [-0.01192], [-0.01336], [0.0052], [-0.01624], [-0.01768], [-0.01912], [-0.02056], [-0.022], [-0.02344], [-0.00488], [-0.00632], [-0.02776], [-0.0292], [0.00936], [-0.01208], [-0.03352], [0.00504], [0.0036], [-0.01784], [-0.01928], [-0.00072], [-0.02216], [-0.0236], [-0.02504], [-0.00648], [-0.00792], [-0.00936], [-0.0308], [-0.01224], [0.00632], [-0.01512], [-0.01656], [-0.018], [-0.01944], [-0.02088], [-0.00232], [-0.00376], [-0.0252], [-0.00664], [-0.00808], [-0.00952], [-0.01096], [0.0076], [-0.01384], [-0.01528], [-0.01672], [0.00184], [0.0004], [-0.00104], [-0.02248], [-0.02392], [-0.02536], [-0.0068], [0.01176], [-0.00968], [-0.01112], [-0.01256], [-0.014], [-0.01544], [0.00312], [-0.01832], [-0.01976], [-0.0212], [-0.00264], [-0.00408], [-0.00552], [-0.02696], [-0.0084], [-0.00984], [0.00872], [-0.03272], [0.00584], [-0.0156], [-0.01704], [-0.01848], [-0.01992], [-0.00136], [-0.0028], [-0.00424], [-0.02568], [-0.00712], [-0.00856], [-0.01], [-0.01144], [-0.01288], [-0.01432], [-0.01576], [-0.0372], [0.00136], [-0.02008], [-0.02152], [-0.02296], [-0.0044], [-0.02584], [-0.00728], [-0.00872], [-0.03016], [-0.0116], [-0.03304], [0.00552], [-0.03592], [-0.01736], [0.0012], [-0.00024], [-0.02168], [-0.02312], [-0.02456], [-0.006], [-0.02744], [-0.00888], [-0.03032], [-0.03176], [-0.0332], [-0.01464], [-0.01608], [-0.01752], [0.00104], [-0.0004], [-0.02184], [-0.00328], [-0.00472], [-0.00616], [-0.0076], [-0.00904], [-0.03048], [-0.01192], [-0.01336], [-0.0148], [-0.01624], [-0.01768], [-0.01912], [-0.02056], [-0.002], [-0.02344], [-0.00488], [-0.00632], [-0.02776], [0.0108], [-0.01064], [-0.01208], [-0.01352], [0.00504], [0.0036], [0.00216], [0.00072], [-0.02072], [-0.02216], [-0.0236], [-0.02504], [-0.00648], [-0.00792], [0.01064], [0.0092], [-0.01224], [-0.01368], [0.00488], [-0.01656], [0.002], [0.00056], [-0.00088], [-0.00232], [-0.00376], [-0.0252], [-0.02664], [-0.00808], [-0.00952], [-0.01096], [-0.0124], [-0.03384], [0.00472], [-0.01672], [-0.01816], [-0.0196], [-0.00104], [-0.00248], [0.01608], [-0.00536], [-0.0068], [-0.00824], [-0.02968], [0.00888], [0.00744], [-0.014], [0.00456], [-0.01688], [0.00168], [-0.01976], [-0.0012], [-0.00264], [-0.00408], [-0.00552], [-0.00696], [-0.0284], [-0.00984], [0.00872], [-0.01272], [-0.01416], [-0.0156], [-0.01704], [-0.01848], [-0.01992], [-0.00136], [-0.0228], [-0.00424], [-0.00568], [-0.00712], [-0.00856], [-0.01], [-0.01144], [-0.01288], [-0.01432], [0.00424], [0.0028], [0.00136], [-0.02008], [-0.00152], [-0.02296], [-0.0044], [-0.00584], [-0.02728], [-0.00872], [-0.03016], [-0.0316], [-0.01304], [0.00552], [-0.03592], [-0.01736], [-0.0188], [-0.00024], [-0.02168], [-0.02312], [0.01544], [-0.006], [-0.00744], [-0.02888], [-0.01032], [-0.01176], [0.0068], [-0.01464], [-0.01608], [-0.01752], [0.00104], [-0.0204], [-0.00184], [-0.00328], [-0.00472], [-0.02616], [-0.0076], [-0.02904], [-0.01048], [-0.01192], [-0.01336], [0.0052], [-0.01624], [-0.01768], [0.00088], [-0.02056], [-0.022], [-0.00344], [-0.02488], [-0.00632], [-0.00776], [-0.0092], [0.00936], [-0.03208], [0.02648], [-0.01496], [0.0036], [-0.01784], [-0.01928], [-0.00072], [-0.00216], [-0.0036], [-0.00504], [-0.00648], [-0.00792], [-0.00936], [0.0092], [-0.03224], [-0.01368], [-0.01512], [-0.01656], [0.002], [-0.01944], [-0.02088], [-0.00232], [-0.00376], [-0.0052], [-0.00664], [-0.00808], [-0.00952], [-0.01096], [-0.0124], [-0.01384], [-0.01528], [-0.01672], [0.00184], [-0.0196], [-0.04104], [-0.02248], [-0.00392], [-0.00536], [-0.0268], [-0.00824], [-0.00968], [-0.01112], [-0.01256], [-0.014], [0.00456], [-0.01688], [-0.01832], [-0.01976], [-0.0012], [-0.02264], [-0.00408], [-0.00552], [0.01304], [0.0116], [-0.00984], [-0.01128], [-0.03272], [-0.01416], [-0.0156], [0.00296], [0.00152], [8e-05], [-0.00136], [-0.0228], [-0.02424], [-0.00568], [-0.00712], [-0.00856], [-0.01], [-0.01144], [0.00712], [0.00568], [0.00424], [-0.0172], [0.00136], [-0.02008], [-0.02152], [-0.02296], [-0.0044], [0.01416], [-0.00728], [-0.02872], [-0.01016], [-0.0316], [-0.01304], [-0.01448], [-0.01592], [-0.01736], [0.0012], [-0.02024], [-0.02168], [-0.00312], [-0.00456], [-0.006], [-0.00744], [0.01112], [-0.03032], [-0.03176], [-0.0332], [-0.01464], [-0.01608], [-0.01752], [0.00104], [-0.0004], [-0.02184], [-0.00328], [0.01528], [-0.02616], [-0.0076], [-0.00904], [-0.01048], [-0.01192], [-0.03336], [-0.0148], [-0.01624], [-0.01768], [0.00088], [-0.02056], [-0.002], [-0.00344], [-0.02488], [-0.02632], [-0.02776], [-0.0092], [-0.01064], [-0.01208], [-0.01352], [-0.01496], [-0.0164], [-0.01784], [0.00072], [-0.00072], [-0.04216], [-0.0236], [-0.00504], [-0.00648], [0.01208], [-0.00936], [-0.0308], [-0.03224], [0.00632], [0.00488], [-0.01656], [0.002], [0.00056], [-0.00088], [-0.02232], [-0.00376], [-0.0052], [-0.00664], [-0.02808], [-0.00952], [-0.01096], [-0.0124], [-0.01384], [-0.01528], [-0.01672], [-0.01816], [0.0004], [-0.02104], [-0.02248], [-0.02392], [-0.02536], [-0.0068], [-0.00824], [-0.00968], [0.00888], [-0.01256], [-0.014], [-0.01544], [0.00312], [-0.03832], [0.00024], [-0.0012], [-0.00264], [-0.02408], [-0.00552], [-0.02696], [-0.0284], [-0.00984], [0.00872], [-0.01272], [-0.01416], [-0.0356], [0.00296], [-0.01848], [8e-05], [-0.00136], [-0.0028], [-0.02424], [-0.02568], [-0.00712], [-0.00856], [-0.01]]
  out "New sawtooth signal":waveform(dbl)(graph)={"t0"=timestamp(0 s since 1904-01-01), "dt"=0.001, "Y"=array[10000 elements]}
  in  "Input will be multiplied by 5":dbl=20.0
  out "Number of Slices":dbl=100.0
  in  "Sawtooth Offset":dbl=0.024 format="%.2p"
  in  "Camera trigger delay (degrees)":dbl=-180.0 format="%.2p"
  in  "Exposure time (ms)":dbl=1000.0
  out "# Samples written per channel":u32=10000
  in  "Stop Analog Signal":bool
  in  "Sawtooth Phase":dbl=180.0 format="%.2p"
  in  "Sawtooth Amplitude":dbl=0.365 format="%.2p"
  in  "Acquire Z Stack?":bool=TRUE
  in  "Z step size (um)":dbl=0.2
  in  "Disable Axis":bool
  out "Error out":errorcluster
  out "Connected":bool=TRUE
  out "GetFirmwareVersion 2":string="3.03\r"
  in  "SPIIPLUSCOM660Lib.IAsyncChannel":refnum<k7>
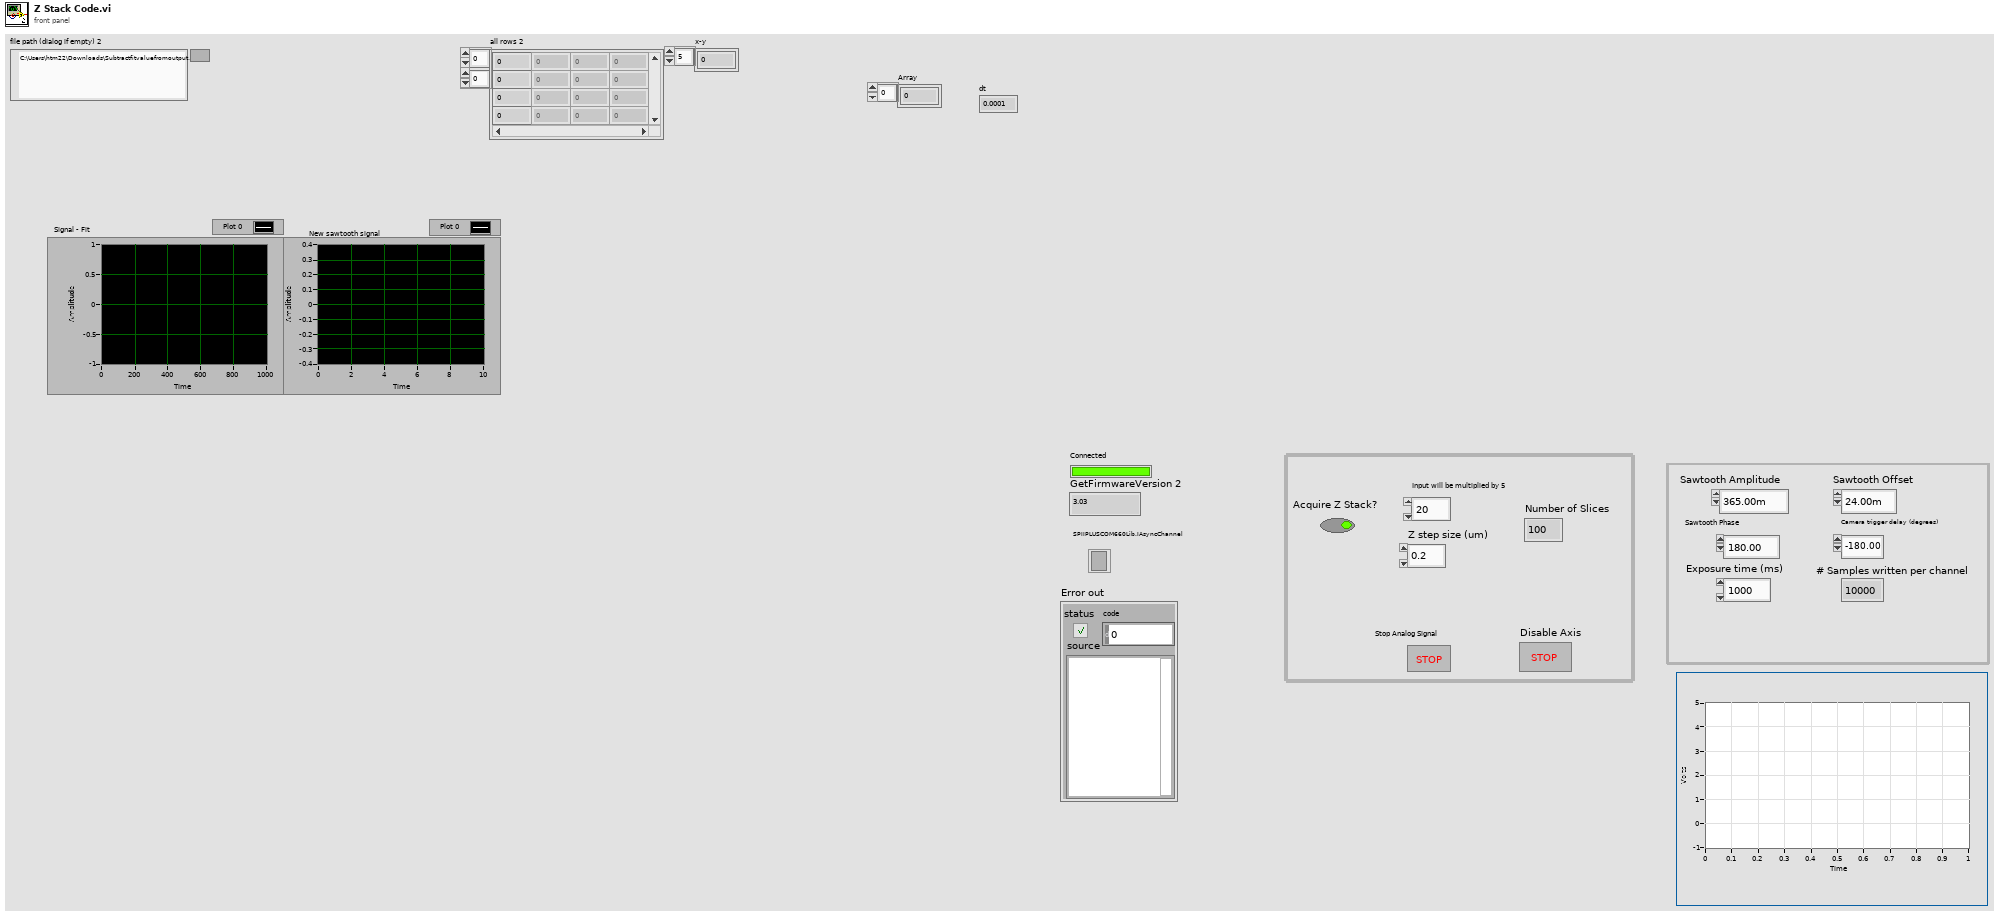
[diagram p1: front panel]
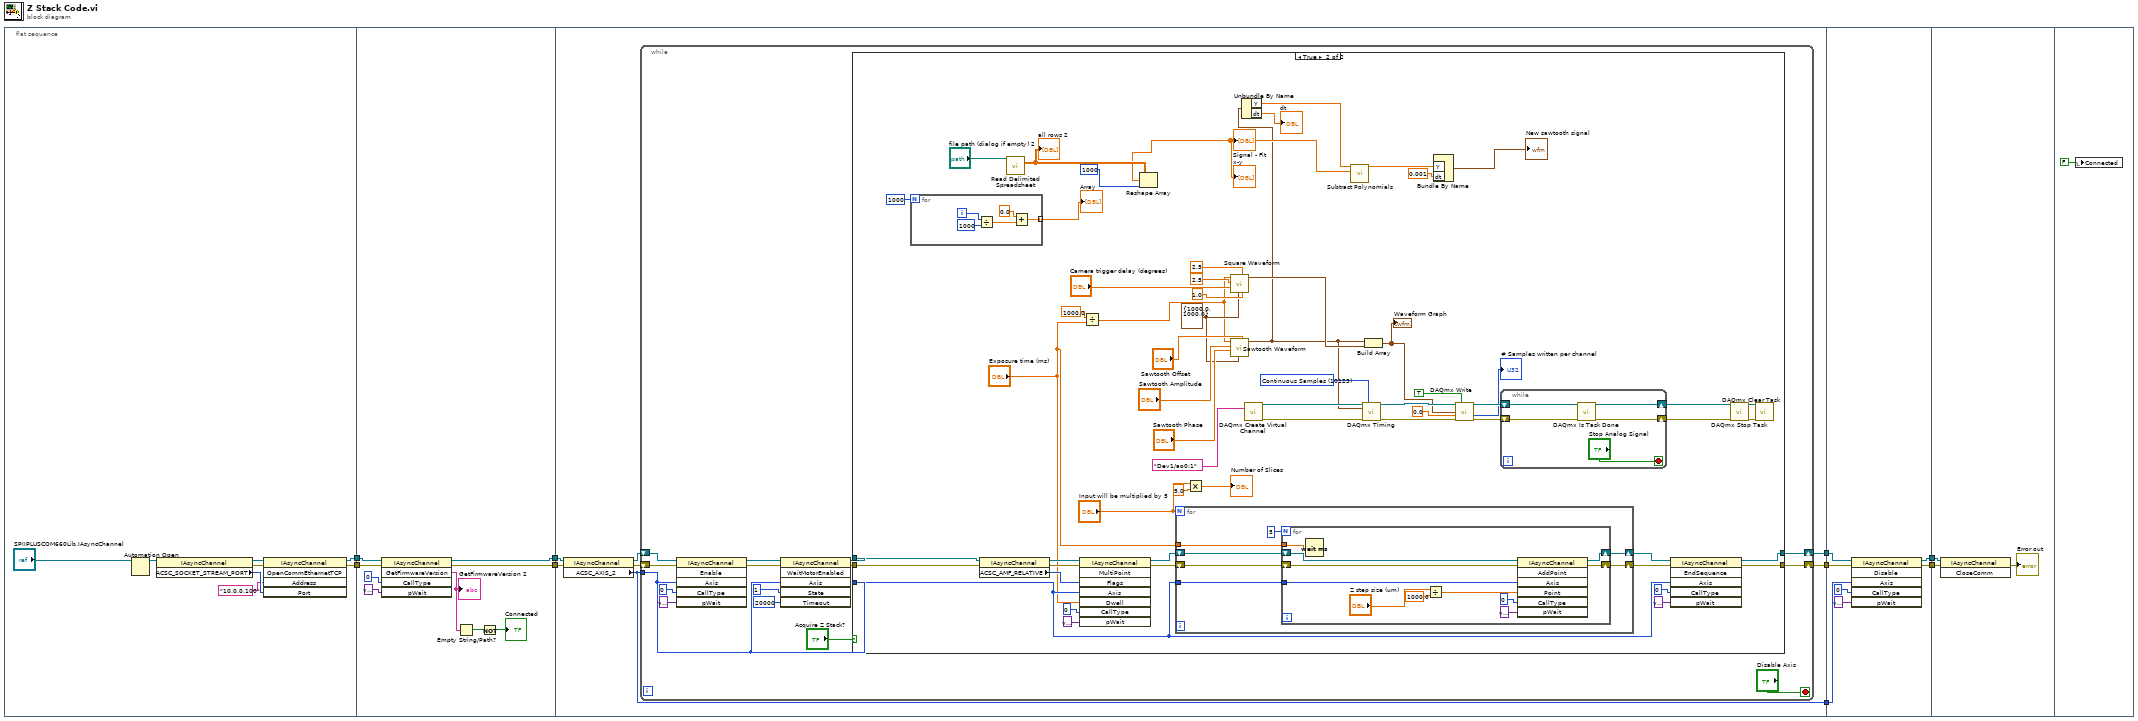
[diagram p0: block diagram]
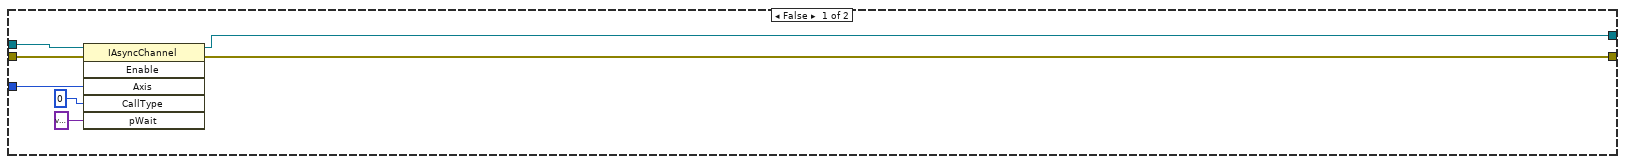
[diagram p2: hidden frame]
diagram:
  n1 = flat-sequence {
    tunnel: [w12] -> w9
    tunnel: [w11] -> w8
    tunnel: w9 -> [w22]
    tunnel: w8 -> [w21]
    tunnel: [w19] -> w7
    tunnel: [w18] -> w6
    tunnel: w7 -> [w31]
    tunnel: w6 -> [w30]
    tunnel: [w33] -> w5
    tunnel: [w32] -> w4
    tunnel: [w29] -> w1
    tunnel: w5 -> [w149]
    tunnel: w4 -> [w148]
    tunnel: [w147] -> w3
    tunnel: [w146] -> w2
    tunnel: w1 -> [w145]
    tunnel: w3 -> [w151]
    tunnel: w2 -> [w150]
    frame #0 {
      n2 = Automation Open(Automation Refnum="SPIIPLUSCOM660Lib.IAsyncChannel") -> (Automation Refnum=w17:refnum<k7>)  [unwired: 3 in, 1 out]
      n3 = property class="IAsyncChannel"(reference=w17) -> (reference out=w16:refnum<k7>, error out=w10:errorcluster, "ACSC_SOCKET_STREAM_PORT"=w14:i32)  [unwired: 1 in]
      n4 = invoke class="IAsyncChannel" method="OpenCommEthernetTCP"(reference=w16, error in=w10, "Address"="10.0.0.100", "Port"=w14) -> (reference out=w12:refnum<k7>, error out=w11:errorcluster)  [unwired: 1 in, 3 out]
    }
    frame #1 {
      n5 = invoke class="IAsyncChannel" method="GetFirmwareVersion"(reference=w22, error in=w21, "CallType"=u64 0, "pWait"=variant) -> (reference out=w19:refnum<k7>, error out=w18:errorcluster, "GetFirmwareVersion"=w24:string)  [unwired: 1 in, 2 out]
      "GetFirmwareVersion 2" <- w24
      n6 = Empty String/Path?(string/path=w24) -> (empty?=w23:bool)
      n7 = Not(x=w23) -> (.not. x?=→"Connected":bool)
    }
    frame #2 {
      n8 = property class="IAsyncChannel"(reference=w31, error in=w30) -> (reference out=w28:refnum<k7>, error out=w27:errorcluster, "ACSC_AXIS_2"=w29:i32)
      n9 = while {
        shift-right: [w48] -> w33
        shift-left: w28 -> [w40]
        shift-right: [w47] -> w32
        shift-left: w27 -> [w39]
        tunnel: w29 -> [w36]
        stop <- "Disable Axis" stop-if-true
        n10 = invoke class="IAsyncChannel" method="Enable"(reference=w40, error in=w39, "Axis"=w36, "CallType"=u64 0, "pWait"=variant) -> (reference out=w44:refnum<k7>, error out=w43:errorcluster)  [unwired: 1 in, 4 out]
        n11 = invoke class="IAsyncChannel" method="WaitMotorEnabled"(reference=w44, error in=w43, "Axis"=w36, "State"=1, "Timeout"=20000) -> (reference out=w35:refnum<k7>, error out=w34:errorcluster)  [unwired: 1 in, 4 out]
        n12 = case shown="True" "Acquire Z Stack?" {
          tunnel: w35 -> [w55 w77]
          tunnel: w34 -> [w54 w78]
          tunnel: [w53 w75] -> w48
          tunnel: [w52 w76] -> w47
          tunnel: w36 -> [w51 w74]
          frame False {
            n13 = invoke class="IAsyncChannel" method="Enable"(reference=w55, error in=w54, "Axis"=w51, "CallType"=u64 0, "pWait"=variant) -> (reference out=w53:refnum<k7>, error out=w52:errorcluster)  [unwired: 1 in, 4 out]
          }
          frame True {
            w90 = cluster{"Fs":dbl, "#s":dbl} {"Fs"=1000.0, "#s"=1000.0} ("sampling info")
            w108 = 10123 items=["Finite Samples"=10178, "Continuous Samples"=10123, "Hardware Timed Single Point"=12522] ("sample mode")
            n14 = for {
              N: 1000 -> [_]
              tunnel: [w115] -> w69 mode=indexing
              i -> [w119]
              n15 = Divide(x=w119, y=1000) -> (x/y=w116:dbl)
              n16 = Add(x=0.0, y=w116) -> (x+y=w115:dbl)
            }
            "Array" <- w69
            n17 = property class="IAsyncChannel"(reference=w77, error in=w78) -> (reference out=w87:refnum<k7>, error out=w86:errorcluster, "ACSC_AMF_RELATIVE"=w83:i32)
            n18 = call-poly <vilib>:"Read Delimited Spreadsheet.vi"("file path (dialog if empty)"="file path (dialog if empty) 2") -> ("all rows"=w63:dbl[][])  [unwired: 9 in, 5 out]
            "all rows 2" <- w63
            n19 = invoke class="IAsyncChannel" method="MultiPoint"(reference=w87, error in=w86, "Flags"=w83, "Axis"=w74, "Dwell"="Exposure time (ms)", "CallType"=u64 0, "pWait"=variant) -> (reference out=w82:refnum<k7>, error out=w81:errorcluster)  [unwired: 1 in, 6 out]
            n20 = Divide(x=1000.0, y="Exposure time (ms)") -> (x/y=w58:dbl)
            n21 = Reshape Array(w63, 1000 ("dimension size")) -> (w61:dbl[])
            "Signal - Fit" <- w61
            "x-y" <- w61
            n22 = for {
              N: "Input will be multiplied by 5" -> [_]
              tunnel: w74 -> [w122]
              tunnel: "Exposure time (ms)" -> [w121]
              shift-right: [w124] -> w80
              shift-left: w82 -> [w126]
              shift-right: [w123] -> w79
              shift-left: w81 -> [w125]
              n23 = for {
                N: 5 -> [_]
                tunnel: w122 -> [w137]
                shift-right: [w132] -> w124
                shift-left: w126 -> [w136]
                shift-right: [w131] -> w123
                shift-left: w125 -> [w135]
                tunnel: w121 -> [w127]
                n24 = Wait (ms)(milliseconds to wait=w127) -> ()  [unwired: 1 out]
                n25 = Divide(x="Z step size (um)", y=1000.0) -> (x/y=w128:dbl)
                n26 = invoke class="IAsyncChannel" method="AddPoint"(reference=w136, error in=w135, "Axis"=w137, "Point"=w128, "CallType"=u64 0, "pWait"=variant) -> (reference out=w132:refnum<k7>, error out=w131:errorcluster)  [unwired: 1 in, 5 out]
              }
            }
            n27 = Multiply(x="Input will be multiplied by 5", y=5.0) -> (x*y=→"Number of Slices":dbl)
            n28 = call <vilib>:"Square Waveform.vi"("duty cycle (%)"=1.0, "offset"=2.5, "sampling info"=w90, "phase"="Camera trigger delay (degrees)", "amplitude"=2.5, "frequency"=w58) -> ("signal out"=w93:waveform(dbl))  [unwired: 4 in, 1 out]
            n29 = call <vilib>:"Sawtooth Waveform.vi"("offset"="Sawtooth Offset", "sampling info"=w90, "phase"="Sawtooth Phase", "amplitude"="Sawtooth Amplitude", "frequency"=w58) -> ("signal out"=w59:waveform(dbl))  [unwired: 5 in, 1 out]
            n30 = Unbundle By Name(w59) -> ("Y"=w66:dbl[], "dt"=→"dt":dbl)
            n31 = call-poly <vilib>:"DAQmx Create Virtual Channel.vi"("physical channels"=tag "Dev1/ao0:1") -> ("task out"=w110:refnum<k21>, "error out"=w109:errorcluster)  [unwired: 13 in]
            n32 = call-poly <vilib>:"Subtract Polynomials.vi"("Q(x)"=w61, "P(x)"=w66) -> ("P(x)-Q(x)"=w67:dbl[])  [unwired: 8 in, 1 out]
            n33 = call-poly <vilib>:"DAQmx Timing.vi"("task/channels in"=w110, "sample mode"=w108, "waveform"=w59, "error in"=w109) -> ("task out"=w105:refnum<k21>, "error out"=w104:errorcluster)  [unwired: 10 in]
            n34 = Build Array(w59, w93) -> (w57:waveform(dbl)[])
            "Waveform Graph" <- w57
            n35 = Bundle By Name("Y"=w67, "dt"=0.001) -> (→"New sawtooth signal":waveform(dbl))  [unwired: 1 in]
            n36 = call-poly <vilib>:"DAQmx Write.vi"("task/channels in"=w105, "auto start"=TRUE, "data"=w57, "timeout"=0.0, "error in"=w104) -> ("task out"=w106:refnum<k21>, "number of samples written per channel"=→"# Samples written per channel":u32, "error out"=w107:errorcluster)  [unwired: 8 in]
            n37 = while {
              shift-right: [w139] -> w101
              shift-left: w106 -> [w142]
              shift-right: [w140] -> w102
              shift-left: w107 -> [w141]
              stop <- "Stop Analog Signal" stop-if-true
              n38 = call <vilib>:"DAQmx Is Task Done.vi"("task/channels in"=w142, "error in"=w141) -> ("task out"=w139:refnum<k21>, "error out"=w140:errorcluster)  [unwired: 11 in, 1 out]
            }
            n39 = invoke class="IAsyncChannel" method="EndSequence"(reference=w80, error in=w79, "Axis"=w74, "CallType"=u64 0, "pWait"=variant) -> (reference out=w75:refnum<k7>, error out=w76:errorcluster)  [unwired: 1 in, 4 out]
            n40 = call <vilib>:"DAQmx Stop Task.vi"("task/channels in"=w101, "error in"=w102) -> ("task out"=w111:refnum<k21>, "error out"=w112:errorcluster)  [unwired: 12 in]
            n41 = call <vilib>:"DAQmx Clear Task.vi"("task in"=w111, "error in"=w112) -> ()  [unwired: 13 in, 1 out]
          }
        }
      }
    }
    frame #3 {
      n42 = invoke class="IAsyncChannel" method="Disable"(reference=w149, error in=w148, "Axis"=w145, "CallType"=u64 0, "pWait"=variant) -> (reference out=w147:refnum<k7>, error out=w146:errorcluster)  [unwired: 1 in, 4 out]
    }
    frame #4 {
      n43 = invoke class="IAsyncChannel" method="CloseComm"(reference=w151, error in=w150) -> (error out=→"Error out":errorcluster)  [unwired: 1 in, 2 out]
    }
    frame #5 {
      n44 = local write "Connected"(FALSE ("Connected")) -> ()
    }
  }
